vi "generateSignalByCase.vi"(0 "ControlCase":T2 items=["00 - Promedio Inicial", "01 - Genera señal aleatoria", "02 - Incrementa t0", "03 - Promedia buen t0", "04 - Inicializa Amplitud", "05 - Incrementa Amplitud", "06 - Promedia buena Amplitud", "07 - Inicializa Sigma", "08 - Incrementa Sigma", "09 - Promedia buen Sigma", "10 - Actualiza mejor señal", "11 - Control ON, Ajuste OFF", "12 - Control OFF"], 1 "Reset Control":bool, 5 "Señal de Control IN":dbl[](array[numeric]), 7 "Sound Parameters":cluster{"# samples":u32, "tiempos (ms)":dbl}, 9 "Parametros Maximos":T1, 11 "detla Parametros":T1) -> (4 "Arreglo de Salida":dbl[](array[numeric]), 6 "Señal de Control OUT":dbl[](array[numeric]), 8 "Parametros Actuales":T1, 15 "Parametros Iniciales":T1)   [LabVIEW 2010]
uses:
  CaseControl.ctl
panel:
  in  "Mejores Parametros IN":T1
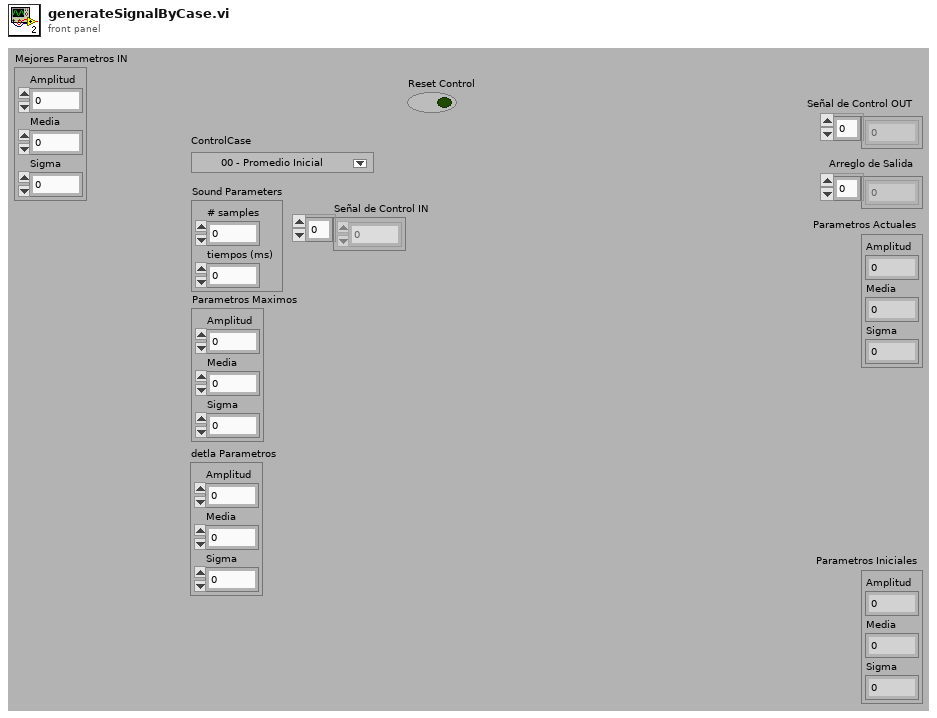
[diagram p1: front panel]
types:
  T1 = cluster{"Amplitud":dbl, "Media":dbl, "Sigma":dbl}
  T2 = typedef "CaseControl.ctl" = u32
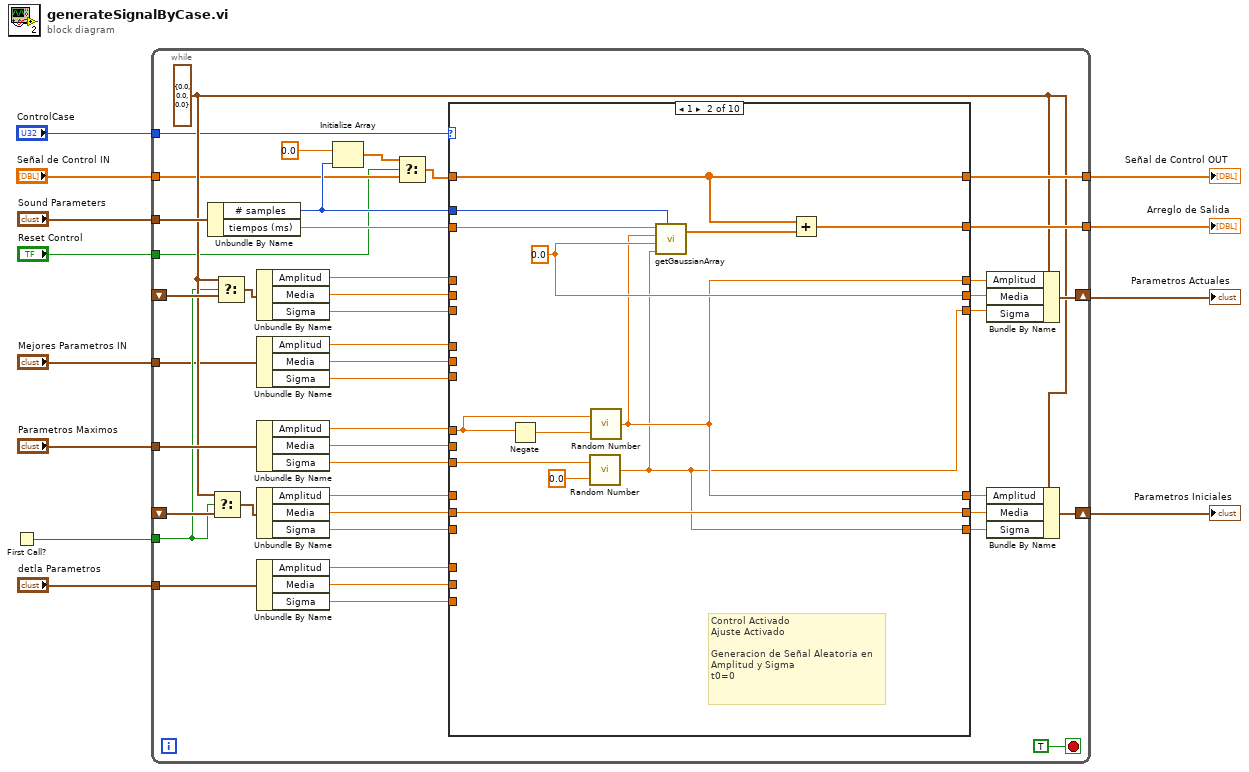
[diagram p0: block diagram]
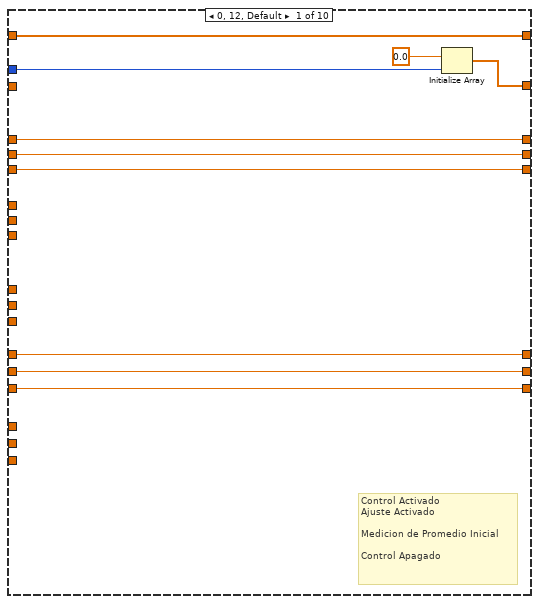
[diagram p2: hidden frame]
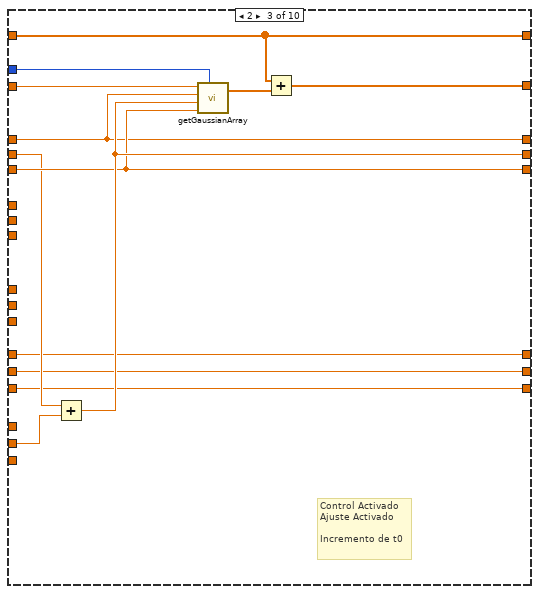
[diagram p3: hidden frame]
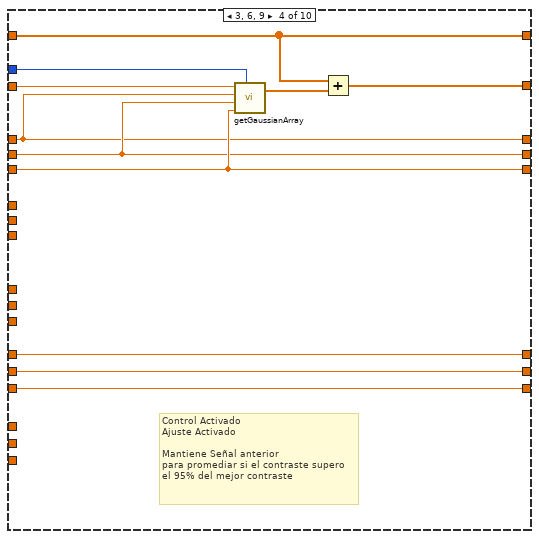
[diagram p4: hidden frame]
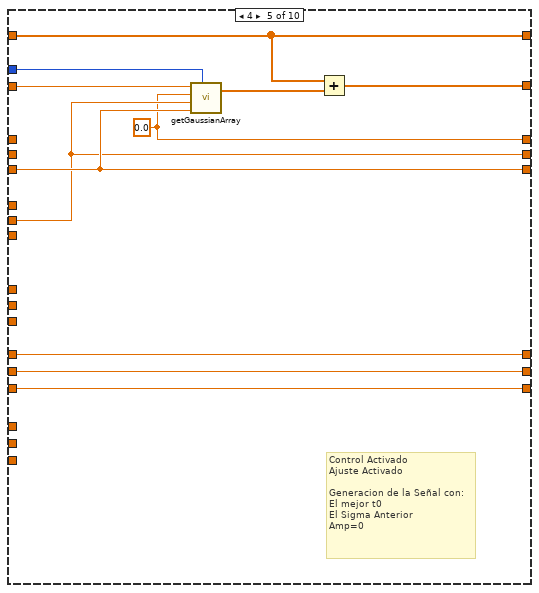
[diagram p5: hidden frame]
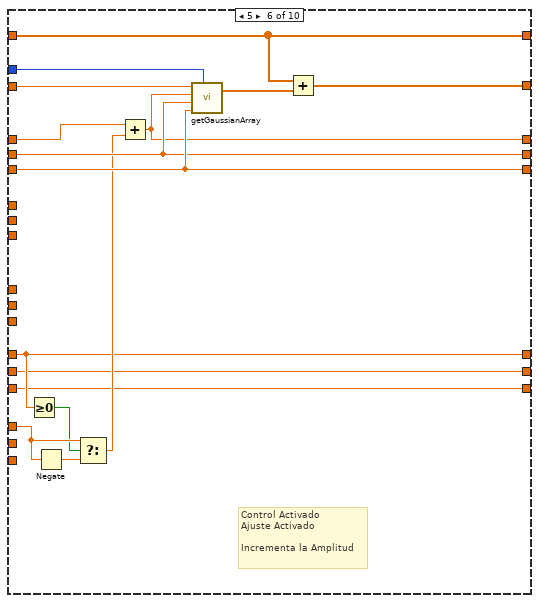
[diagram p6: hidden frame]
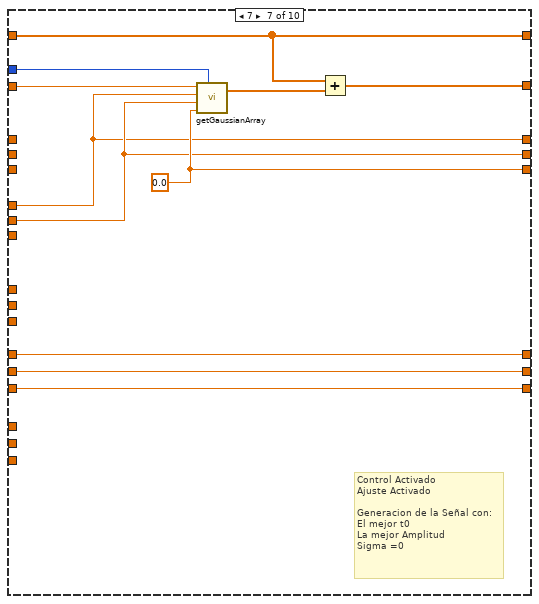
[diagram p7: hidden frame]
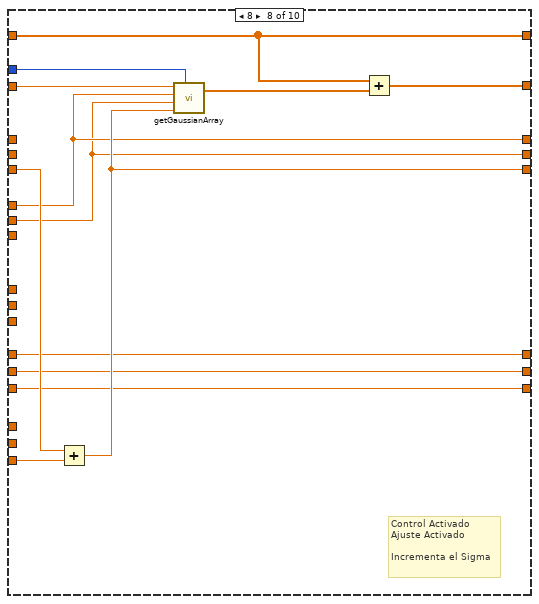
[diagram p8: hidden frame]
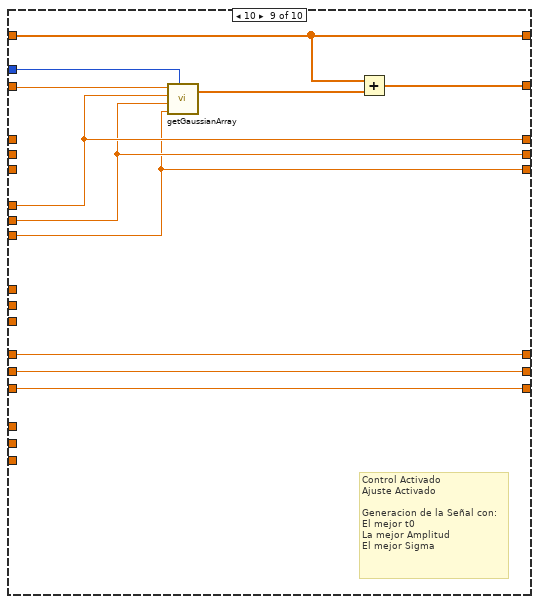
[diagram p9: hidden frame]
diagram:
  n1 = First Call?() -> (First Call?: T/F=w6:bool)
  n2 = while {
    tunnel: [w55] -> w11
    tunnel: "detla Parametros" -> [w52]
    tunnel: "Parametros Maximos" -> [w48]
    tunnel: "Sound Parameters" -> [w37]
    shift-right: [w30] -> w5
    shift-left: _ -> [w25]
    tunnel: w6 -> [w16]
    shift-right: [w43] -> w8
    shift-left: _ -> [w24]
    tunnel: "Reset Control" -> [w14]
    tunnel: "ControlCase" -> [w15]
    tunnel: "Señal de Control IN" -> [w19]
    tunnel: [w56] -> w12
    tunnel: "Mejores Parametros IN" -> [w13]
    stop <- TRUE stop-if-true
    w23 = T1 {"Amplitud"=0.0, "Media"=0.0, "Sigma"=0.0} ("input cluster")
    n3 = Unbundle By Name(w37) -> ("# samples"=w20:u32, "tiempos (ms)"=w36:dbl)
    n4 = Select(t=w23, s=w16, f=w25) -> (s? t:f=w26:T1)
    n5 = Select(t=w23, s=w16, f=w24) -> (s? t:f=w22:T1)
    n6 = Unbundle By Name(w22) -> ("Amplitud"=w40:dbl, "Media"=w42:dbl, "Sigma"=w41:dbl)
    n7 = Unbundle By Name(w13) -> ("Amplitud"=w54:dbl, "Media"=w53:dbl, "Sigma"=w38:dbl)
    n8 = Unbundle By Name(w48) -> ("Amplitud"=w47:dbl, "Media"=w39:dbl, "Sigma"=w46:dbl)
    n9 = Unbundle By Name(w26) -> ("Amplitud"=w33:dbl, "Media"=w32:dbl, "Sigma"=w31:dbl)
    n10 = Unbundle By Name(w52) -> ("Amplitud"=w51:dbl, "Media"=w50:dbl, "Sigma"=w49:dbl)
    n11 = Initialize Array(0.0 ("element"), w20) -> (w18:dbl[])
    n12 = Select(t=w18, s=w14, f=w19) -> (s? t:f=w17:dbl[])
    n13 = case shown="1" w15 {
      tunnel: [w65 w75 w90 w103 w114 w130 w140 w154 w155 w172] -> w55
      tunnel: w20 -> [w66 w70 w87 w97 w109 w115 w133 w150 w161 _]
      tunnel: w36 -> [_ w71 w86 w98 w108 w116 w134 w149 w160 _]
      tunnel: w47 -> [_ w78 _ _ _ _ _ _ _ _]
      tunnel: w46 -> [_ w77 _ _ _ _ _ _ _ _]
      tunnel: [w58 w72 w92 w101 w110 w128 w132 w145 w158 w171] -> w35
      tunnel: [w60 w68 w85 w96 w107 w117 w131 w146 w159 w169] -> w45
      tunnel: [w57 w67 w91 w102 w113 w129 w141 w153 w157 w170] -> w44
      tunnel: w50 -> [_ _ w84 _ _ _ _ _ _ _]
      tunnel: w42 -> [w58 _ w83 w101 _ w128 _ _ _ w171]
      tunnel: w41 -> [w57 _ w91 w102 w113 w129 _ w148 _ w170]
      tunnel: w40 -> [w60 _ w85 w96 _ w125 _ _ _ w169]
      tunnel: w17 -> [w61 w73 w88 w99 w111 w126 w136 w152 w156 w172]
      tunnel: [w61 w73 w88 w99 w111 w126 w136 w152 w156 w172] -> w56
      tunnel: w53 -> [_ _ _ _ w110 _ w132 w145 w158 _]
      tunnel: w54 -> [_ _ _ _ _ _ w131 w146 w159 _]
      tunnel: w51 -> [_ _ _ _ _ w123 _ _ _ _]
      tunnel: w49 -> [_ _ _ _ _ _ _ w147 _ _]
      tunnel: w38 -> [_ _ _ _ _ _ _ _ w157 _]
      tunnel: w39 -> [_ _ _ _ _ _ _ _ _ _]
      tunnel: w33 -> [w64 _ w82 w95 w106 w120 w139 w144 w165 w168]
      tunnel: w32 -> [w63 w69 w81 w94 w105 w119 w138 w143 w164 w167]
      tunnel: w31 -> [w62 _ w80 w93 w104 w118 w137 w142 w163 w166]
      tunnel: [w64 w68 w82 w95 w106 w120 w139 w144 w165 w168] -> w29
      tunnel: [w63 w69 w81 w94 w105 w119 w138 w143 w164 w167] -> w28
      tunnel: [w62 w67 w80 w93 w104 w118 w137 w142 w163 w166] -> w27
      frame 0, 12, Default {
        # "Control Activado\nAjuste Activado\n\nMedicion de Promedio Inicial\n\nControl Apagado"
        n14 = Initialize Array(0.0, w66) -> (w65:dbl[])
      }
      frame 1 {
        w72 = 0.0 ("t0 (ms)")
        # "Control Activado\nAjuste Activado\n\nGeneracion de Señal Aleatoria en\nAmplitud y Sigma\nt0=0"
        n15 = Negate(x=w78) -> (-x=w79:dbl)
        n16 = call "Random Number.vi"("Min"=0.0, "Max"=w77) -> ("Out"=w67:dbl)
        n17 = call "Random Number.vi"("Min"=w79, "Max"=w78) -> ("Out"=w68:dbl)
        n18 = call "getGaussianArray.vi"("tiempo (ms)"=w71, "Amplitud"=w68, "t0 (ms)"=w72, "Sigma (ms)"=w67, "#samples"=w70) -> ("Y out"=w74:dbl[])  [unwired: 1 out]
        n19 = Add(x=w73, y=w74) -> (x+y=w75:dbl[])
      }
      frame 2 {
        # "Control Activado\nAjuste Activado\n\nIncremento de t0"
        n20 = Add(x=w83, y=w84) -> (x+y=w92:dbl)
        n21 = call "getGaussianArray.vi"("tiempo (ms)"=w86, "Amplitud"=w85, "t0 (ms)"=w92, "Sigma (ms)"=w91, "#samples"=w87) -> ("Y out"=w89:dbl[])  [unwired: 1 out]
        n22 = Add(x=w88, y=w89) -> (x+y=w90:dbl[])
      }
      frame 3, 6, 9 {
        # "Control Activado\nAjuste Activado\n\nMantiene Señal anterior \npara promediar si el contraste supero\nel 95% del mejor contraste"
        n23 = call "getGaussianArray.vi"("tiempo (ms)"=w98, "Amplitud"=w96, "t0 (ms)"=w101, "Sigma (ms)"=w102, "#samples"=w97) -> ("Y out"=w100:dbl[])  [unwired: 1 out]
        n24 = Add(x=w99, y=w100) -> (x+y=w103:dbl[])
      }
      frame 4 {
        w107 = 0.0 ("Amplitud")
        # "Control Activado\nAjuste Activado\n\nGeneracion de la Señal con:\nEl mejor t0\nEl Sigma Anterior\nAmp=0"
        n25 = call "getGaussianArray.vi"("tiempo (ms)"=w108, "Amplitud"=w107, "t0 (ms)"=w110, "Sigma (ms)"=w113, "#samples"=w109) -> ("Y out"=w112:dbl[])  [unwired: 1 out]
        n26 = Add(x=w111, y=w112) -> (x+y=w114:dbl[])
      }
      frame 5 {
        # "Control Activado\nAjuste Activado\n\nIncrementa la Amplitud"
        n27 = Greater Or Equal To 0?(x=w120) -> (x >= 0?=w122:bool)
        n28 = Negate(x=w123) -> (-x=w124:dbl)
        n29 = Select(t=w123, s=w122, f=w124) -> (s? t:f=w121:dbl)
        n30 = Add(x=w125, y=w121) -> (x+y=w117:dbl)
        n31 = call "getGaussianArray.vi"("tiempo (ms)"=w116, "Amplitud"=w117, "t0 (ms)"=w128, "Sigma (ms)"=w129, "#samples"=w115) -> ("Y out"=w127:dbl[])  [unwired: 1 out]
        n32 = Add(x=w126, y=w127) -> (x+y=w130:dbl[])
      }
      frame 7 {
        w141 = 0.0 ("Sigma (ms)")
        # "Control Activado\nAjuste Activado\n\nGeneracion de la Señal con:\nEl mejor t0\nLa mejor Amplitud\nSigma =0"
        n33 = call "getGaussianArray.vi"("tiempo (ms)"=w134, "Amplitud"=w131, "t0 (ms)"=w132, "Sigma (ms)"=w141, "#samples"=w133) -> ("Y out"=w135:dbl[])  [unwired: 1 out]
        n34 = Add(x=w136, y=w135) -> (x+y=w140:dbl[])
      }
      frame 8 {
        # "Control Activado\nAjuste Activado\n\nIncrementa el Sigma"
        n35 = Add(x=w148, y=w147) -> (x+y=w153:dbl)
        n36 = call "getGaussianArray.vi"("tiempo (ms)"=w149, "Amplitud"=w146, "t0 (ms)"=w145, "Sigma (ms)"=w153, "#samples"=w150) -> ("Y out"=w151:dbl[])  [unwired: 1 out]
        n37 = Add(x=w152, y=w151) -> (x+y=w154:dbl[])
      }
      frame 10 {
        # "Control Activado\nAjuste Activado\n\nGeneracion de la Señal con:\nEl mejor t0\nLa mejor Amplitud\nEl mejor Sigma"
        n38 = call "getGaussianArray.vi"("tiempo (ms)"=w160, "Amplitud"=w159, "t0 (ms)"=w158, "Sigma (ms)"=w157, "#samples"=w161) -> ("Y out"=w162:dbl[])  [unwired: 1 out]
        n39 = Add(x=w156, y=w162) -> (x+y=w155:dbl[])
      }
      frame 11 {
        # "Control Activado\nAjuste desactivado"
      }
    }
    n40 = Bundle By Name(cluster=w23, "Amplitud"=w45, "Media"=w35, "Sigma"=w44) -> (w43:T1)
    n41 = Bundle By Name(cluster=w23, "Amplitud"=w29, "Media"=w28, "Sigma"=w27) -> (w30:T1)
  }
  "Señal de Control OUT" <- w12
  "Arreglo de Salida" <- w11
  "Parametros Actuales" <- w8
  "Parametros Iniciales" <- w5
